vi "read_params.vi"(8 "error in (no error)":errorcluster, 11 "MiniBatchSparsePCA in":refnum<class "MiniBatchSparsePCA.lvclass">) -> (0 "error out":errorcluster, 2 "params":T1={"n_components"={"n_components_type"="None", "n_components_int"=0.0}, "alpha"=1.0, "ridge_alpha"=0.01, "n_iter"=100.0, "batch_size"=3.0, "verbose"=0.0, "shuffle"=TRUE, "n_jobs"=1.0, "method"="lars", "random_state"=0.0}, 3 "MiniBatchSparsePCA out":refnum<class "MiniBatchSparsePCA.lvclass">)   [LabVIEW 2020, in "MiniBatchSparsePCA.lvclass"]
uses:
  MiniBatchSparsePCA.lvclass
  Controls/mini_batch_sparse_pca_params.ctl
  MiniBatchSparsePCA.lvclass/MiniBatchSparsePCA.ctl
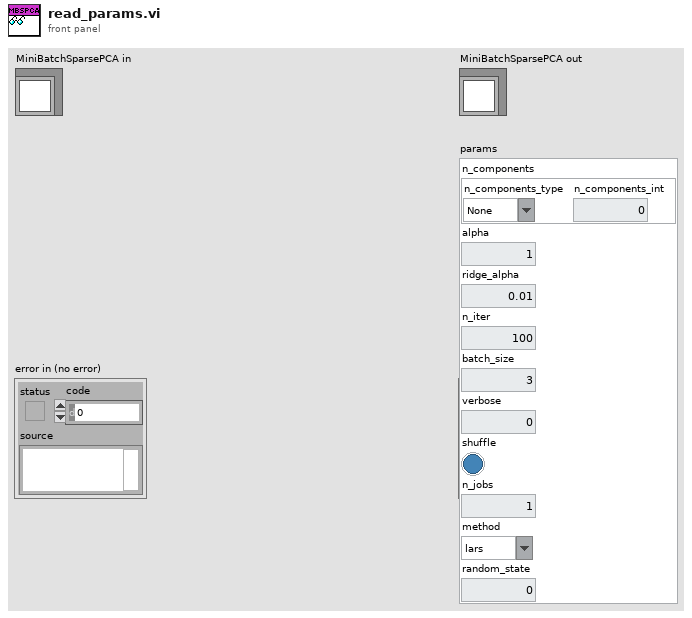
[diagram p1: front panel]
types:
  T1 = typedef "mini_batch_sparse_pca_params.ctl" = cluster{"n_components":cluster{"n_components_type":string, "n_components_int":dbl}, "alpha":dbl, "ridge_alpha":dbl, "n_iter":dbl, "batch_size":dbl, "verbose":dbl, "shuffle":bool, "n_jobs":dbl, "method":string, "random_state":dbl}
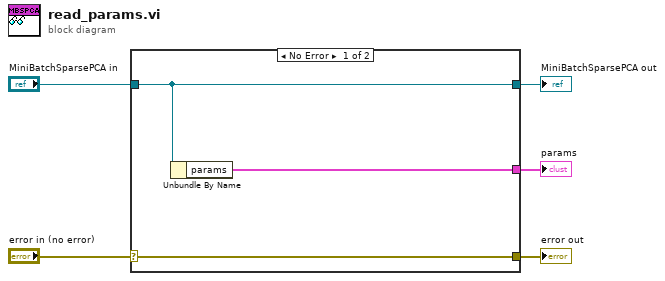
[diagram p0: block diagram]
diagram:
  n1 = case shown="No Error" "error in (no error)" {
    selector: "error in (no error)" -> [w8 w9]
    tunnel: [w8 w9] -> w4
    tunnel: [w7 w10] -> w2
    tunnel: "MiniBatchSparsePCA in" -> [w7 w10]
    tunnel: [w6 _] -> w1
    frame No Error {
      n2 = Unbundle By Name(w7) -> ("params"=w6:T1)
    }
    frame Error {
    }
  }
  "error out" <- w4
  "MiniBatchSparsePCA out" <- w2
  "params" <- w1
